vi "Get Velocity from Motors.vi"   [LabVIEW 2017, in "NI_Robotics_Steering Frame.lvclass"]
doc: "Calculates the steering frame velocity or arc velocity required to best satisfy the velocity and angle of each motor. You must manually select the polymorphic instance to use."
uses:
  <vilib>/robotics/Steering/Steering Frame/NI_Robotics_Steering Frame.lvclass
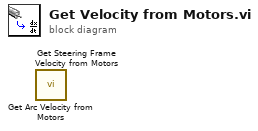
[diagram p0: block diagram]
diagram:
  n1 = call <vilib>:"Get Arc Velocity from Motors.vi"() -> ()  [unwired: 9 in, 3 out]
  n2 = call <vilib>:"Get Steering Frame Velocity from Motors.vi"() -> ()  [unwired: 9 in, 3 out]
